vi "Swerve Drive 6181.vi"(0 "X":dbl(slide) scale=-1.0..1.0, 1 "Y":dbl(slide) scale=1.0..-1.0, 2 "Z":dbl(knob) scale=1.0..-1.0, 3 "Robot-Centric":bool, 4 "Auto Controls":bool) -> ()   [LabVIEW 2019]
uses:
  <vilib>/Rock Robotics/Network Tables/NT Write Number.vi
panel:
  in  "Robot Length":dbl=21.5
  in  "Robot Width":dbl=29.5
  # "SWERVE DRIVE\nVersion 3.1\n\nCory Lynch\nApple Pi Robotics\nTeam 2067"
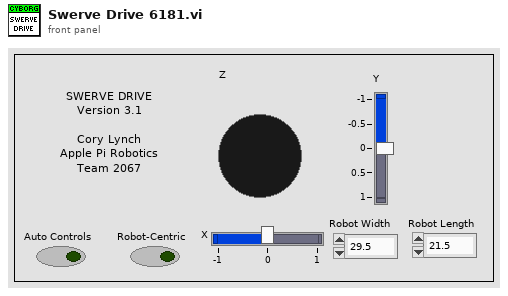
[diagram p1: front panel]
types:
  T1 = enum16{"Back Left", "Back Right", "Front Left", "Front Right"}
  T2 = cluster{"Yaw":dbl, "Roll":dbl, "Pitch":dbl, "Heading":dbl, "Fused Heading":dbl}
  T3 = typedef "WPI_MotorControlDeviceRef.ctl" = cluster{"DeviceStatus":errorcluster, "Type":T4, "PWM":cluster{"PWM Channel":T5, "DeadBand":T6}, "CAN":cluster{"Device Number":u8, "SetOutput VI Ref":variant, "GetOutput VI Ref":variant, "Enable VI Ref":variant, "Disable VI Ref":variant, "Data":variant}, "Invert":bool, "DIO PWM":cluster{"PWM \"Enable\" Channel":T5, "DIOChannel":T7, "PWM Rate":dbl}}
  T4 = typedef "WPI_MotorControlType.ctl" = enum16{"PWM", "CAN", "DIO PWM"}
  T5 = typedef "FPGA_DIOPWMChannel.ctl" = enum8{"PWM 0", "PWM 1", "PWM 2", "PWM 3", "PWM 4", "PWM 5", "PWM 6", "PWM 7", "PWM 8", "PWM 9", "PWM MXP 0", "PWM MXP 1", "PWM MXP 2", "PWM MXP 3", "PWM MXP 4", "PWM MXP 5", "PWM MXP 6", "PWM MXP 7", "PWM MXP 8", "PWM MXP 9", "Invalid"}
  T6 = typedef "WPI_PWMDeadband.ctl" = cluster{"Name":string, "maxPositivePwm":i32, "minPositivePwm":i32, "centerPwm":i32, "maxNegativePwm":i32, "minNegativePwm":i32, "angularRange":u16}
  T7 = typedef "FPGA_DIOChannel.ctl" = enum8{"DIO 0", "DIO 1", "DIO 2", "DIO 3", "DIO 4", "DIO 5", "DIO 6", "DIO 7", "DIO 8", "DIO 9", "DIO MXP 0", "DIO MXP 1", "DIO MXP 2", "DIO MXP 3", "DIO MXP 4", "DIO MXP 5", "DIO MXP 6", "DIO MXP 7", "DIO MXP 8", "DIO MXP 9", "DIO MXP 10", "DIO MXP 11", "DIO MXP 12", "DIO MXP 13", "DIO MXP 14", "DIO MXP 15", "SPI Port CS1", "SPI Port CS2", "SPI Port CS3", "SPI Port MISO", "SPI Port MOSI", "Invalid"}
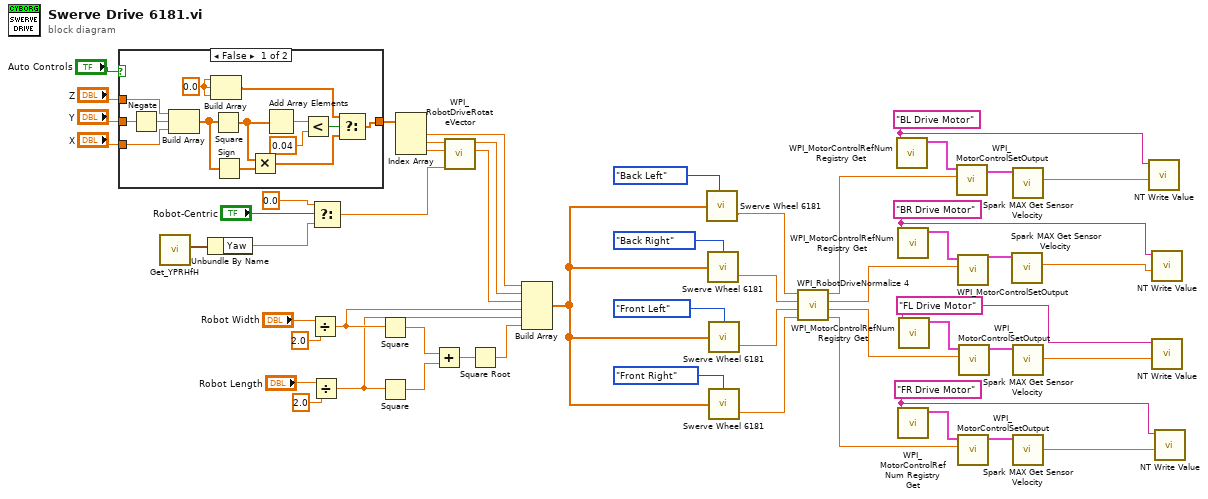
[diagram p0: block diagram]
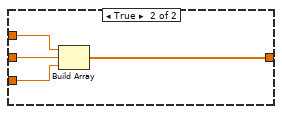
[diagram p2: hidden frame]
diagram:
  w2 = "FR Drive Motor" ("refnum name")
  w4 = "FL Drive Motor" ("refnum name")
  w5 = "BR Drive Motor" ("refnum name")
  w7 = "BL Drive Motor" ("refnum name")
  n1 = case shown="False" "Auto Controls" {
    tunnel: "Y" -> [w65 w71]
    tunnel: "X" -> [w59 w72]
    tunnel: "Z" -> [w55 w69]
    tunnel: [w56 w70] -> w34
    frame False {
      w63 = 0.0 ("element")
      n2 = Negate(x=w65) -> (-x=w58:dbl)
      n3 = Build Array(w55, w58, w59) -> (w62:dbl[])
      n4 = Build Array(w63, w63, w63) -> (w64:dbl[])
      n5 = Square(x=w62) -> (x^2=w60:dbl[])
      n6 = Sign(1:w62) -> (0:w61:dbl[])
      n7 = Multiply(x=w60, y=w61) -> (x*y=w57:dbl[])
      n8 = Add Array Elements(numeric array=w60) -> (sum=w68:dbl)
      n9 = Less?(x=w68, y=0.04 ("x")) -> (x < y?=w66:bool)
      n10 = Select(t=w64, s=w66, f=w57) -> (s? t:f=w56:dbl[])
    }
    frame True {
      n11 = Build Array(w69, w71, w72) -> (w70:dbl[])
    }
  }
  n12 = call <vilib>:"Get_YPRHfH.vi"() -> ("YRPHfH"=w25:T2)  [unwired: 11 in]
  n13 = Unbundle By Name(w25) -> ("Yaw"=w26:dbl)
  n14 = Divide(x="Robot Width", y=2.0) -> (x/y=w24:dbl)
  n15 = Divide(x="Robot Length", y=2.0) -> (x/y=w23:dbl)
  n16 = Select(t=0.0, s="Robot-Centric", f=w26) -> (s? t:f=w31:dbl)
  n17 = Square(x=w24) -> (x^2=w44:dbl)
  n18 = Square(x=w23) -> (x^2=w45:dbl)
  n19 = Index Array(array=w34) -> (element #1=w30:dbl, element #2=w35:dbl, element #3=w38:dbl)  [unwired: 3 in]
  n20 = Add(x=w44, y=w45) -> (x+y=w43:dbl)
  n21 = call <vilib>:"WPI_RobotDriveRotateVector.vi"("Angle"=w31, "X"=w38, "Y"=w35) -> ("X'"=w33:dbl, "Y'"=w29:dbl)  [unwired: 7 out]
  n22 = Square Root(x=w43) -> (sqrt(x)=w22:dbl)
  n23 = Build Array(w30, w29, w33, w24, w23, w22) -> (w14:dbl[])
  n24 = call "Swerve Wheel 6181.vi"("Wheel"=T1."Back Left", "Inputs"=w14) -> ("Speed"=w21:dbl)  [unwired: 3 in]
  n25 = call "Swerve Wheel 6181.vi"("Wheel"=T1."Back Right", "Inputs"=w14) -> ("Speed"=w19:dbl)  [unwired: 3 in]
  n26 = call "Swerve Wheel 6181.vi"("Wheel"=T1."Front Left", "Inputs"=w14) -> ("Speed"=w17:dbl)  [unwired: 3 in]
  n27 = call "Swerve Wheel 6181.vi"("Wheel"=T1."Front Right", "Inputs"=w14) -> ("Speed"=w15:dbl)  [unwired: 3 in]
  n28 = call <vilib>:"WPI_RobotDriveNormalize 4.vi"("D"=w15, "C"=w17, "B"=w19, "A"=w21) -> ("D'"=w47:dbl, "C'"=w48:dbl, "B'"=w49:dbl, "A'"=w50:dbl)
  n29 = call <vilib>:"WPI_MotorControlRefNum Registry Get.vi"("refnum name"=w7) -> ("MotorControlDevRef"=w54:T3)  [unwired: 9 in, 1 out]
  n30 = call <vilib>:"WPI_MotorControlRefNum Registry Get.vi"("refnum name"=w5) -> ("MotorControlDevRef"=w53:T3)  [unwired: 9 in, 1 out]
  n31 = call <vilib>:"WPI_MotorControlRefNum Registry Get.vi"("refnum name"=w2) -> ("MotorControlDevRef"=w51:T3)  [unwired: 9 in, 1 out]
  n32 = call <vilib>:"WPI_MotorControlRefNum Registry Get.vi"("refnum name"=w4) -> ("MotorControlDevRef"=w52:T3)  [unwired: 9 in, 1 out]
  n33 = call <vilib>:"WPI_MotorControlSetOutput.vi"("Output"=w50, "MotorControlDevRef"=w54) -> ("MotorControlDevRef"=w12:T3)  [unwired: 7 in, 2 out]
  n34 = call <vilib>:"WPI_MotorControlSetOutput.vi"("Output"=w49, "MotorControlDevRef"=w53) -> ("MotorControlDevRef"=w11:T3)  [unwired: 7 in, 2 out]
  n35 = call <vilib>:"WPI_MotorControlSetOutput.vi"("Output"=w47, "MotorControlDevRef"=w51) -> ("MotorControlDevRef"=w9:T3)  [unwired: 7 in, 2 out]
  n36 = call <vilib>:"WPI_MotorControlSetOutput.vi"("Output"=w48, "MotorControlDevRef"=w52) -> ("MotorControlDevRef"=w10:T3)  [unwired: 7 in, 2 out]
  n37 = call <vilib>:"Spark MAX Get Sensor Velocity.vi"("MotorControlDevRef in"=w11) -> ("Sensor Velocity"=w6:dbl)  [unwired: 7 in, 3 out]
  n38 = call <vilib>:"Spark MAX Get Sensor Velocity.vi"("MotorControlDevRef in"=w12) -> ("Sensor Velocity"=w8:dbl)  [unwired: 7 in, 3 out]
  n39 = call <vilib>:"Spark MAX Get Sensor Velocity.vi"("MotorControlDevRef in"=w10) -> ("Sensor Velocity"=w3:dbl)  [unwired: 7 in, 3 out]
  n40 = call <vilib>:"Spark MAX Get Sensor Velocity.vi"("MotorControlDevRef in"=w9) -> ("Sensor Velocity"=w1:dbl)  [unwired: 7 in, 3 out]
  n41 = call-poly <vilib>:"NT Write Value.vi"("Numeric"=w8, "Name"=w7) -> ()  [unwired: 9 in, 1 out]
  n42 = call-poly <vilib>:"NT Write Value.vi"("Numeric"=w6, "Name"=w5) -> ()  [unwired: 9 in, 1 out]
  n43 = call-poly <vilib>:"NT Write Value.vi"("Numeric"=w3, "Name"=w4) -> ()  [unwired: 9 in, 1 out]
  n44 = call-poly <vilib>:"NT Write Value.vi"("Numeric"=w1, "Name"=w2) -> ()  [unwired: 9 in, 1 out]
